vi "Hide Animated Busy Icon with Message and Abort Button.vi"(2 "Already active? (F)":bool, 3 "Message":string, 7 "Target VI reference":refnum<vi>, 11 "Error In":errorcluster, 16 "Abort Button Name (Abort)":string="Abort", 17 "Animated Busy Icon Control Name (Animated Busy Icon)":string="Animated Busy Icon", 18 "Message Control Name (Message)":string="Message") -> (10 "Error Out":errorcluster)   [LabVIEW 2021, in "GUI.lvlib"]
doc: "This VI passes error in through and ignores it."
uses:
  GUI/GUI.lvlib
  Utilities/Utilities.lvlib
  Error/Error.lvlib
panel:
  # "see the License on the block diagram (Ctrl+E or Window:Show Block Diagram)"
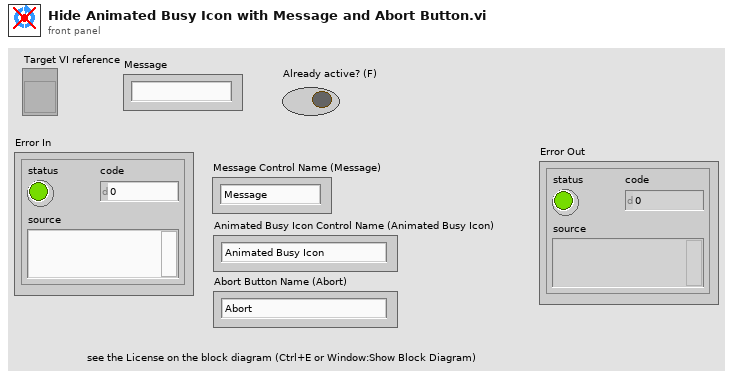
[diagram p1: front panel]
types:
  T1 = enum16{"Controls & Indicators", "Controls", "Indicators"}
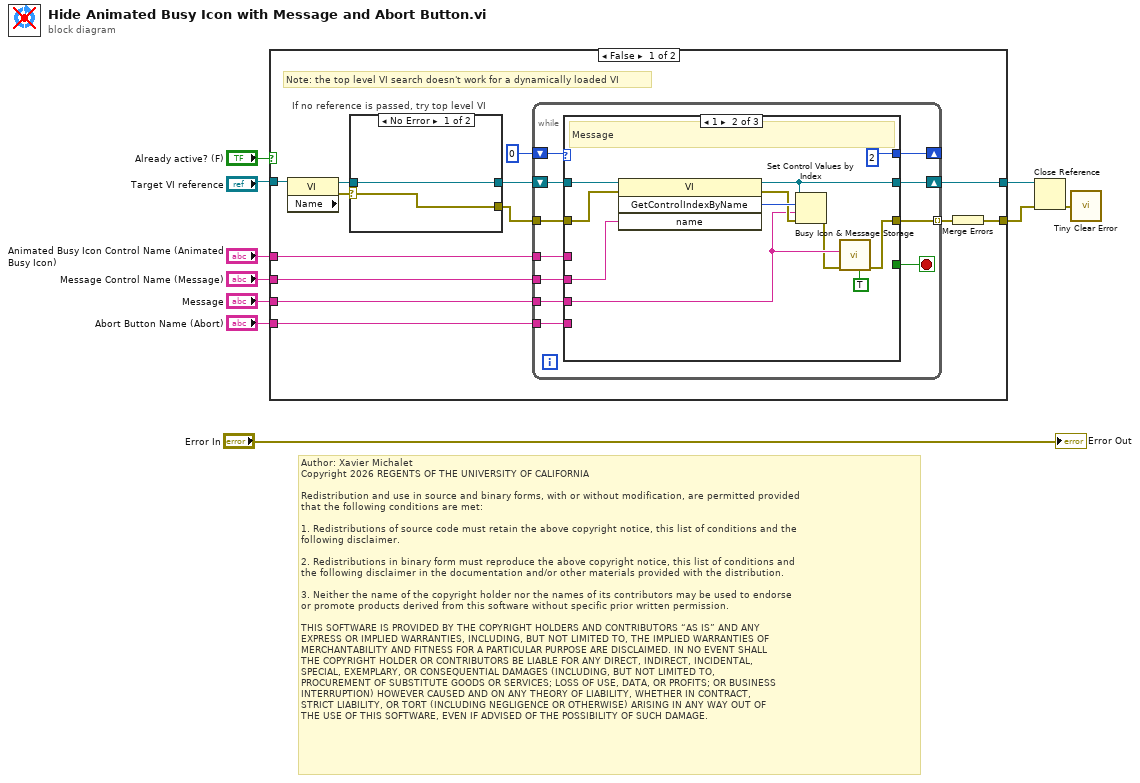
[diagram p0: block diagram]
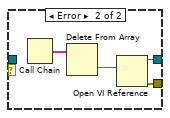
[diagram p2: hidden frame]
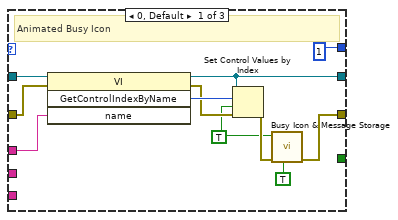
[diagram p3: hidden frame]
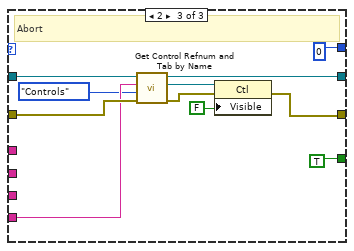
[diagram p4: hidden frame]
diagram:
  # "Author: Xavier Michalet\nCopyright 2026 REGENTS OF THE UNIVERSITY OF CALIFORNIA\n\nRedistribution and use in source and binary forms, with or without modification, are permitted provided\nthat the following conditions are met:\n\n1. Redistributions of source code must retain the above copyright notice, this list of conditions and the\nfollowing disclaimer.\n\n2. Redistributions in binary form must reproduce the above copyright notice, this list of conditions and\nthe following disclaimer in the documentation and/or other materials provided with the distribution.\n\n3. Neither the name of the copyright holder nor the names of its contributors may be used to endorse \nor promote products derived from this software without specific prior written permission.\n\nTHIS SOFTWARE IS PROVIDED BY THE COPYRIGHT HOLDERS AND CONTRIBUTORS “AS IS” AND ANY \nEXPRESS OR IMPLIED WARRANTIES, INCLUDING, BUT NOT LIMITED TO, THE IMPLIED WARRANTIES OF\nMERCHANTABILITY AND FITNESS FOR A PARTICULAR PURPOSE ARE DISCLAIMED. IN NO EVENT SHALL\nTHE COPYRIGHT HOLDER OR CONTRIBUTORS BE LIABLE FOR ANY DIRECT, INDIRECT, INCIDENTAL, \nSPECIAL, EXEMPLARY, OR CONSEQUENTIAL DAMAGES (INCLUDING, BUT NOT LIMITED TO, \nPROCUREMENT OF SUBSTITUTE GOODS OR SERVICES; LOSS OF USE, DATA, OR PROFITS; OR BUSINESS\nINTERRUPTION) HOWEVER CAUSED AND ON ANY THEORY OF LIABILITY, WHETHER IN CONTRACT, \nSTRICT LIABILITY, OR TORT (INCLUDING NEGLIGENCE OR OTHERWISE) ARISING IN ANY WAY OUT OF\nTHE USE OF THIS SOFTWARE, EVEN IF ADVISED OF THE POSSIBILITY OF SUCH DAMAGE."
  n1 = case shown="False" "Already active? (F)" {
    tunnel: [w23 w74] -> w10
    tunnel: [w11 _] -> w9
    tunnel: "Message Control Name (Message)" -> [w20 _]
    tunnel: "Animated Busy Icon Control Name (Animated Busy Icon)" -> [w19 _]
    tunnel: "Message" -> [w18 _]
    tunnel: "Target VI reference" -> [w15 w74]
    tunnel: "Abort Button Name (Abort)" -> [w12 _]
    frame False {
      # "Note: the top level VI search doesn't work for a dynamically loaded VI"
      n2 = property class="VI" props=["Name"](reference=w15) -> (reference out=w14:refnum<vi>, error out=w13:errorcluster)  [unwired: 1 in, 1 out]
      n3 = case "If no reference is passed, try top level VI" shown="No Error" w13 {
        selector: w13 -> [w24 _]
        tunnel: [w24 w29] -> w16
        tunnel: [w25 w28] -> w17
        tunnel: w14 -> [w25 _]
        frame No Error {
        }
        frame Error {
          n4 = Call Chain() -> (call chain=w26:string[])
          n5 = Delete From Array(array=w26) -> (deleted portion=w27:string)  [unwired: 2 in, 1 out]
          n6 = Open VI Reference(vi path=w27) -> (vi reference=w28:refnum<vi>, error out=w29:errorcluster)  [unwired: 5 in]
        }
      }
      n7 = while {
        shift-right: [w38] -> w23
        shift-left: w17 -> [w39]
        shift-right: [w35] -> _
        shift-left: 0 -> [w36]
        tunnel: w20 -> [w33]
        tunnel: w19 -> [w32]
        tunnel: w18 -> [w31]
        tunnel: w12 -> [w30]
        tunnel: w16 -> [w40]
        tunnel: [w37] -> w22 mode=indexing
        stop <- w34 stop-if-true
        n8 = case shown="1" w36 {
          tunnel: w40 -> [w49 w60 w68]
          tunnel: w39 -> [w48 w59 w69]
          tunnel: [w47 w58 w66] -> w38
          tunnel: [w43 w53 w64] -> w37
          tunnel: [1 2 0] -> w35
          tunnel: [_ _ TRUE] -> w34
          tunnel: w33 -> [_ w56 _]
          tunnel: w32 -> [w45 _ _]
          tunnel: w31 -> [_ w55 _]
          tunnel: w30 -> [_ _ w67]
          frame 0, Default {
            w42 = TRUE ("Visible")
            # "Animated Busy Icon"
            n9 = invoke class="VI" method="GetControlIndexByName"(reference=w48, error in=w49, "name"=w45) -> (reference out=w47:refnum<vi>, error out=w50:errorcluster, "GetControlIndexByName"=w51:i32)  [unwired: 1 in, 1 out]
            n10 = Set Control Values by Index(0:w47, 1:w51, 2:w42, 3:w50) -> (11:w44:errorcluster)
            n11 = call "Busy Icon & Message Storage.vi"("Get(F)/Set Busy Icon"=TRUE, "Error In"=w44, "Busy Icon Status (F = busy)"=w42) -> ("Error Out"=w43:errorcluster)  [unwired: 6 in, 2 out]
          }
          frame 1 {
            # "Message"
            n12 = invoke class="VI" method="GetControlIndexByName"(reference=w59, error in=w60, "name"=w56) -> (reference out=w58:refnum<vi>, error out=w61:errorcluster, "GetControlIndexByName"=w62:i32)  [unwired: 1 in, 1 out]
            n13 = Set Control Values by Index(0:w58, 1:w62, 2:w55, 3:w61) -> (11:w54:errorcluster)
            n14 = call "Busy Icon & Message Storage.vi"("Get(F)/Set Message"=TRUE, "Error In"=w54, "Message String"=w55) -> ("Error Out"=w53:errorcluster)  [unwired: 6 in, 2 out]
          }
          frame 2 {
            # "Abort"
            n15 = call "Get Control Refnum and Tab by Name.vi"("error in"=w68, "Selection"=T1."Controls", "Control Label"=w67, "VI  Ref"=w69) -> ("error out"=w70:errorcluster, "Ctl Refnum"=w71:refnum<vi>, "VI  Ref (dup)"=w66:refnum<vi>)  [unwired: 3 in, 2 out]
            n16 = property class="Ctl"(reference=w71, error in=w70, "Visible"=FALSE) -> (error out=w64:errorcluster)  [unwired: 1 out]
          }
        }
      }
      n17 = Merge Errors(w22) -> (w11:errorcluster)
    }
    frame True {
    }
  }
  n18 = Close Reference(reference=w10, error in (no error)=w9) -> (error out=w1:errorcluster)
  n19 = call "Tiny Clear Error.vi"("Error In"=w1) -> ()  [unwired: 8 in, 1 out]
  "Error Out" <- "Error In"
